vi "synnax channel retrive keys.vi"(7 "handle":u64, 8 "error in (no error)":errorcluster, 10 "count":u64, 11 "name(s)":string) -> (0 "error out":errorcluster, 2 "out_dtypes":string[](array[numeric]), 3 "out_keys":u32[](array[numeric]))   [LabVIEW 2026, in "synnax_clib.lvlib" / "Synnax Client.lvclass"]
uses:
  Synnax Client.lvclass
  synnax_clib.lvlib
  synnax_clib.dll
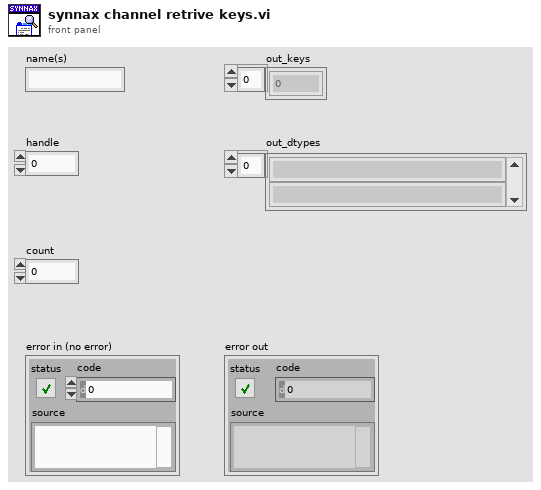
[diagram p1: front panel]
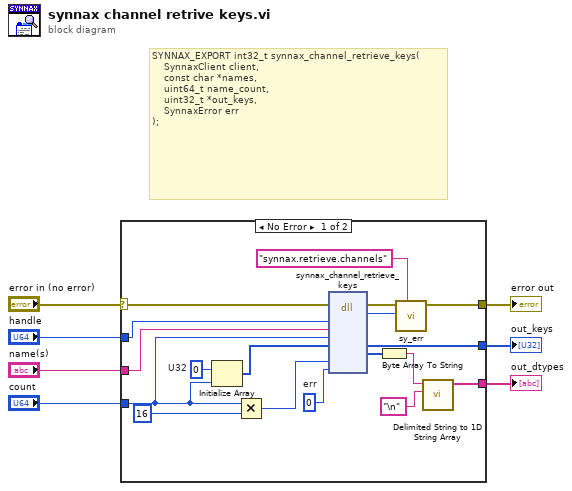
[diagram p0: block diagram]
diagram:
  # "SYNNAX_EXPORT int32_t synnax_channel_retrieve_keys(\n    SynnaxClient client,\n    const char *names,\n    uint64_t name_count,\n    uint32_t *out_keys,\n    SynnaxError err\n);"
  n1 = case shown="No Error" "error in (no error)" {
    selector: "error in (no error)" -> [w13 w26]
    tunnel: "handle" -> [w25 _]
    tunnel: "name(s)" -> [w24 _]
    tunnel: [w23 _] -> w5
    tunnel: [w19 w26] -> w4
    tunnel: "count" -> [w11 _]
    tunnel: [w15 _] -> w2
    frame No Error {
      w12 = u32 0  # U32
      w22 = u64 0  # err
      n2 = Initialize Array(w12, w11) -> (w10:u32[])
      n3 = Multiply(x=w11, y=u64 16) -> (x*y=w17:u64)
      n4 = dll-call lib="C/synnax/client/labview/synnax_clib.*" fn="synnax_channel_retrieve_keys"(error in=w13, "client"=w25, "names"=w24, "name_count"=w11, "out_keys"=w10, "out_dtypes_size"=w17, "err"=w22) -> (error out=w20:errorcluster, "return type"=w18:i32, "out_keys"=w23:u32[], "out_dtypes"=w9:u8[])  [unwired: 8 in, 1 out]
      n5 = Byte Array To String(unsigned byte array=w9) -> (string=w8:string)
      n6 = call "sy_err.vi"("source"="synnax.retrieve.channels", "error code"=w18, "error in (no error)"=w20) -> ("error out"=w19:errorcluster)  [unwired: 8 in]
      n7 = call <vilib>:"Delimited String to 1D String Array.vi"("delimiter"="\n", "delimited string"=w8) -> ("string array"=w15:string[])  [unwired: 9 in]
    }
    frame Error {
    }
  }
  "out_keys" <- w5
  "error out" <- w4
  "out_dtypes" <- w2
